vi "_Update DV Values.vi"(9 "UserInput":i32, 11 "FileNames":path[](array[path])) -> (0 "error out":errorcluster)   [LabVIEW 2015]
uses:
  C:/GitRepo/PerkinElmer/QRD-FW-Server/Sniffer.900/External Dependencies/PerkinElmer.SimplicityServer.LVWrapper.dll
  External Dependencies/PerkinElmer.SimplicityServer.LVWrapper.dll
  <userlib>/_OpenG.lib/file/file.llb/Strip Path Extension - String__ogtk.vi
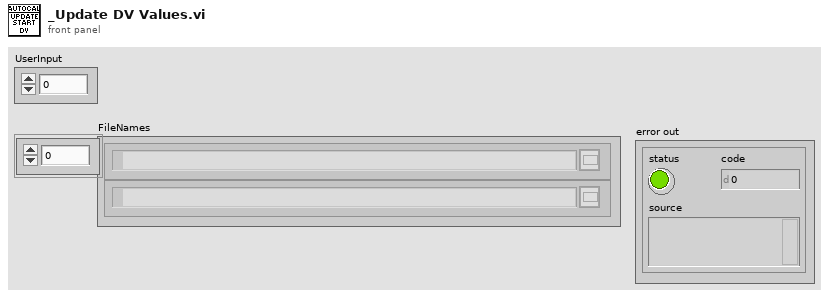
[diagram p1: front panel]
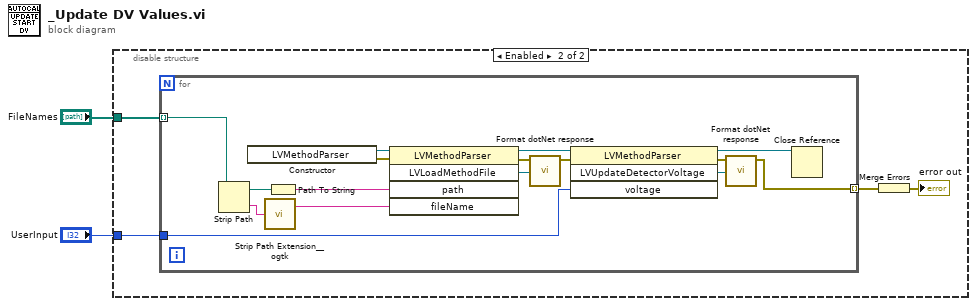
[diagram p0: block diagram]
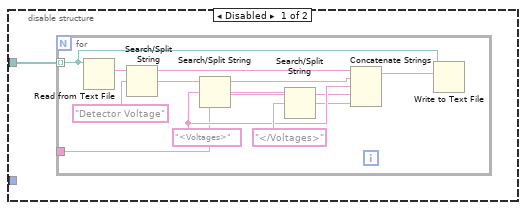
[diagram p2: hidden frame]
diagram:
  n1 = disable-structure shown="Enabled" {
    disable-tunnel: "FileNames" -> [w3 w20]
    disable-tunnel: "UserInput" -> [_ w19]
    frame Disabled {
      n2 = for {
        tunnel: w3 -> [w6] mode=indexing
        tunnel: [w7] -> w4
        w9 = "<Voltages>" ("search string/char (-)")
        n3 = Read from Text File(file (use dialog)=w6) -> (text=w16:string)  [unwired: 3 in, 3 out]
        n4 = Search/Split String(string=w16, search string/char (-)="Detector Voltage") -> (substring before match=w11:string, match + rest of string=w14:string)  [unwired: 1 in, 1 out]
        n5 = Search/Split String(string=w14, search string/char (-)=w9) -> (substring before match=w10:string, match + rest of string=w12:string)  [unwired: 1 in, 1 out]
        n6 = Search/Split String(string=w12, search string/char (-)="</Voltages>") -> (match + rest of string=w8:string)  [unwired: 1 in, 2 out]
        n7 = Concatenate Strings(w11, w10, w9, w7, w8) -> (w5:string)
        n8 = Write to Text File(file (use dialog)=w6, text=w5) -> ()  [unwired: 2 in, 3 out]
      }
    }
    frame Enabled {
      n9 = for {
        tunnel: w20 -> [w32] mode=indexing
        tunnel: w19 -> [w25]
        tunnel: [w21] -> w18 mode=indexing
        n10 = Strip Path(path=w32) -> (stripped path=w34:path, name=w33:string)
        n11 = constructor class="LVMethodParser"() -> (reference out=w35:refnum<k24>, error out=w36:errorcluster)  [unwired: 3 in, 1 out]
        n12 = call-poly <userlib>:"Strip Path Extension__ogtk.vi"("path"=w33) -> ("root"=w30:string)  [unwired: 1 out]
        n13 = Path To String(path=w34) -> (string=w31:string)
        n14 = invoke class="LVMethodParser" method="LVLoadMethodFile"(reference=w35, error in=w36, "path"=w31, "fileName"=w30) -> (reference out=w27:refnum<k24>, error out=w29:errorcluster, "LVLoadMethodFile"=w28:refnum<k24>)  [unwired: 1 in, 2 out]
        n15 = call "Format dotNet response.vi"(".NET Refnum in"=w28, "error in (no error)"=w29) -> ("error IO"=w26:errorcluster)  [unwired: 9 in]
        n16 = invoke class="LVMethodParser" method="LVUpdateDetectorVoltage"(reference=w27, error in=w26, "voltage"=w25) -> (reference out=w22:refnum<k24>, error out=w24:errorcluster, "LVUpdateDetectorVoltage"=w23:refnum<k24>)  [unwired: 1 in, 1 out]
        n17 = call "Format dotNet response.vi"(".NET Refnum in"=w23, "error in (no error)"=w24) -> ("error IO"=w21:errorcluster)  [unwired: 9 in]
        n18 = Close Reference(reference=w22) -> ()  [unwired: 1 in, 1 out]
      }
      n19 = Merge Errors(w18) -> (→"error out":errorcluster)
    }
  }
